vi "Get Active App and Active VI Name.vi"(8 "错误输入（无错误）":errorcluster) -> (0 "错误输出":errorcluster, 2 "应用程序:活动:VI":string, 3 "应用程序:活动:应用程序":refnum<vi>)   [LabVIEW 2012, in "Application.lvlib"]
uses:
  Application.lvlib
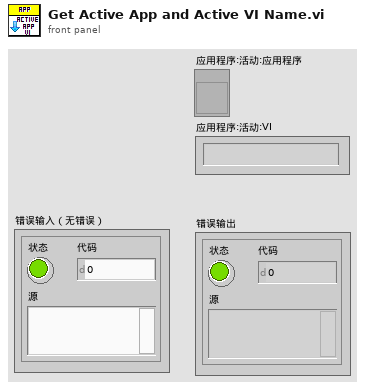
[diagram p1: front panel]
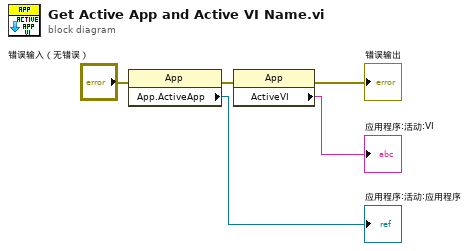
[diagram p0: block diagram]
diagram:
  n1 = property class="App"(error in="错误输入（无错误）") -> (error out=w4:errorcluster, "App.ActiveApp"=→"应用程序:活动:应用程序":refnum<vi>)  [unwired: 1 in, 1 out]
  n2 = property class="App"(error in=w4) -> (error out=→"错误输出":errorcluster, "ActiveVI"=→"应用程序:活动:VI":string)  [unwired: 1 in, 1 out]
